vi "timer.vi"(10 "T_iniz":dbl, 11 "Azione":enum32{"START", "STOP", "RESET", "RIPRENDI"}(ring)) -> (3 "f":dbl)   [LabVIEW 2019]
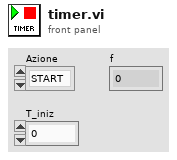
[diagram p1: front panel]
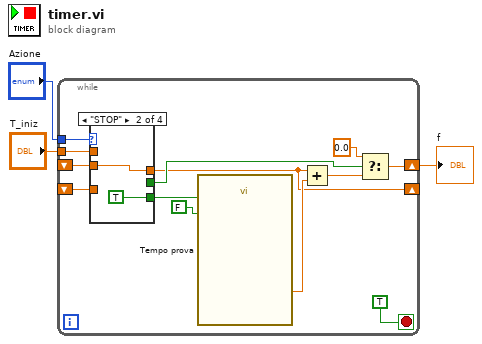
[diagram p0: block diagram]
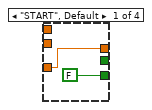
[diagram p2: hidden frame]
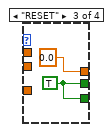
[diagram p3: hidden frame]
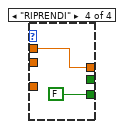
[diagram p4: hidden frame]
diagram:
  n1 = while {
    shift-right: [w5] -> _
    shift-left: _ -> [w12]
    tunnel: "T_iniz" -> [w9]
    tunnel: "Azione" -> [w8]
    shift-right: [w6] -> w1
    shift-left: _ -> [w4]
    stop <- TRUE stop-if-true
    n2 = case shown="\"STOP\"" w8 {
      tunnel: [_ _ w21 _] -> w16
      tunnel: w12 -> [w18 _ _ _]
      tunnel: [w18 w19 0.0 ("f") w24] -> w5
      tunnel: [FALSE TRUE w21 FALSE] -> w11
      tunnel: w9 -> [_ _ _ w24]
      tunnel: w4 -> [_ w19 _ _]
      frame "START", Default {
      }
      frame "STOP" {
      }
      frame "RESET" {
        w21 = TRUE
      }
      frame "RIPRENDI" {
      }
    }
    n3 = call "Tempo prova"("Reset"=w11, "Auto Reset"=FALSE) -> ("Elapsed Time (s)"=w14:dbl)  [unwired: 10 in, 7 out]
    n4 = Add(x=w5, y=w14) -> (x+y=w13:dbl)
    n5 = Select(t=0.0 ("f"), s=w16, f=w13) -> (s? t:f=w6:dbl)
  }
  "f" <- w1
